vi "Update Worker List.vi"(8 "error in (no error)":errorcluster, 11 "BuildServer in":refnum<class "BuildServer.lvclass">) -> (0 "error out":errorcluster, 3 "BuildServer out":refnum<class "BuildServer.lvclass">)   [LabVIEW 2017, in "BuildServer.lvlib" / "BuildServer.lvclass"]
uses:
  BuildServer.lvclass
  BuildServer.lvclass/BuildServer.ctl
  Classes/Comm Interface/Get Msg Update Event.vi
  Classes/Comm Interface/Get Worker Count.vi
  Classes/Comm Interface/Comm Interface.lvclass
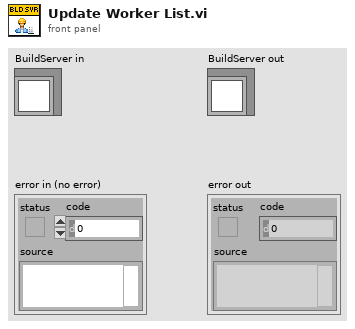
[diagram p1: front panel]
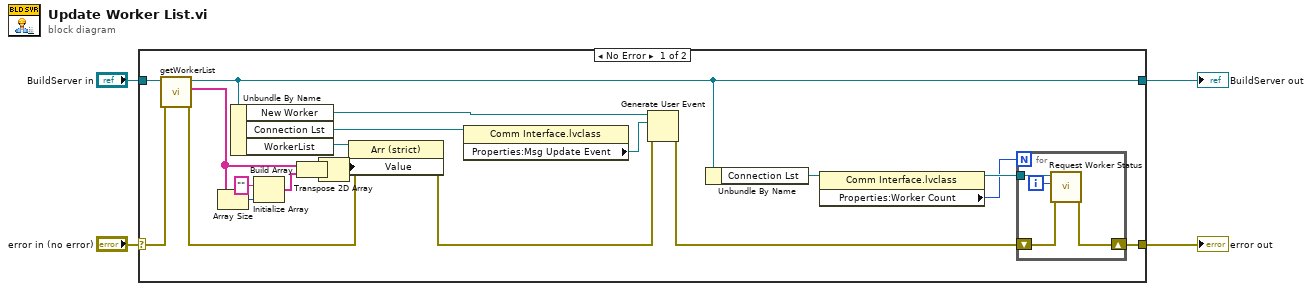
[diagram p0: block diagram]
diagram:
  n1 = case shown="No Error" "error in (no error)" {
    selector: "error in (no error)" -> [w21 w30]
    tunnel: [w5 w30] -> w3
    tunnel: [w7 w29] -> w1
    tunnel: "BuildServer in" -> [w24 w29]
    frame No Error {
      n2 = call "getWorkerList.vi"("error in (no error)"=w21, "BuildServer in"=w24) -> ("error out"=w20:errorcluster, "Worker List"=w13:string[], "BuildServer out"=w7:refnum<class "BuildServer.lvclass">)  [unwired: 7 in]
      n3 = Array Size(array=w13) -> (size(s)=w14:i32)
      n4 = Unbundle By Name(w7) -> ("New Worker"=w18:refnum<user-event>, "Connection Lst"=w19:refnum<class "Comm Interface.lvclass">, "WorkerList"=w23:refnum<vi>)
      n5 = Initialize Array("", w14) -> (w15:string[])
      n6 = Build Array(w13, w15) -> (w22:string[][])
      n7 = Transpose 2D Array(2D array=w22) -> (transposed array=w12:string[][])
      n8 = property class="Arr (strict)"(reference=w23, error in=w20, "Value"=w12) -> (error out=w11:errorcluster)  [unwired: 1 out]
      n9 = property class="Comm Interface.lvclass"(reference=w19) -> ("Properties:Msg Update Event"=w17:refnum<user-event>)  [unwired: 1 in, 2 out]
      n10 = Generate User Event(user event=w18, event data cluster=w17, error in=w11) -> (error out=w6:errorcluster)  [unwired: 1 in, 1 out]
      n11 = Unbundle By Name(w7) -> ("Connection Lst"=w10:refnum<class "Comm Interface.lvclass">)
      n12 = property class="Comm Interface.lvclass"(reference=w10) -> (reference out=w9:refnum<class "Comm Interface.lvclass">, "Properties:Worker Count"=w8:i32)  [unwired: 1 in, 1 out]
      n13 = for {
        N: w8 -> [_]
        tunnel: w9 -> [w28]
        shift-right: [w25] -> w5
        shift-left: w6 -> [w26]
        i -> [w27]
        n14 = call "Request Worker Status.vi"("error in (no error)"=w26, "index"=w27, "Comm Interface in"=w28) -> ("error out"=w25:errorcluster)  [unwired: 7 in, 1 out]
      }
    }
    frame Error {
    }
  }
  "error out" <- w3
  "BuildServer out" <- w1
